vi "DATOS Y GUARDADO.vi"(6 "DATO":string, 8 "error in (no error)":errorcluster, 9 "PROVIENE DE?":enum16{"CONTADOR", "GENERADOR F"}(ring), 10 "Path":path, 11 "GUARDADOTEXTOPLANO in":refnum<class "GUARDADOTEXTOPLANO.lvclass">) -> (0 "error out":errorcluster, 3 "GUARDADOTEXTOPLANO out":refnum<class "GUARDADOTEXTOPLANO.lvclass">)   [LabVIEW 2019, in "GUARDADOTEXTOPLANO.lvlib" / "GUARDADOTEXTOPLANO.lvclass"]
uses:
  GUARDADOTEXTOPLANO.lvclass
  GUARDADOTEXTOPLANO.lvclass/GUARDADOTEXTOPLANO.ctl
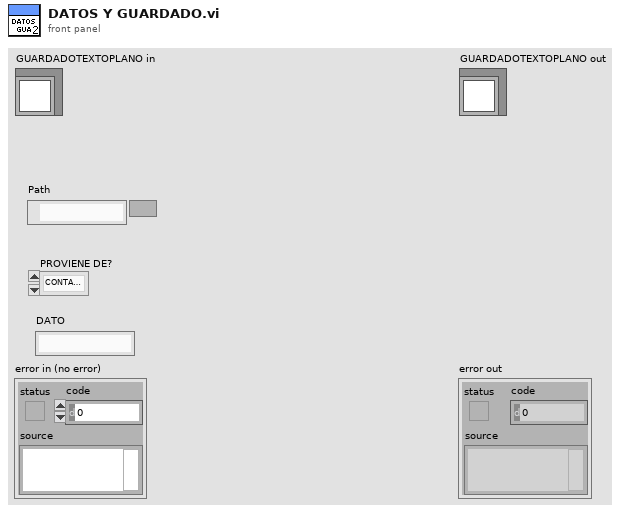
[diagram p1: front panel]
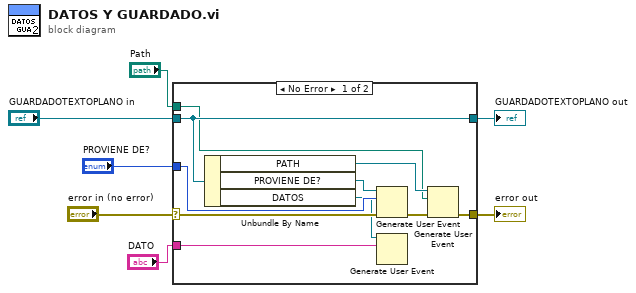
[diagram p0: block diagram]
diagram:
  n1 = case shown="No Error" "error in (no error)" {
    selector: "error in (no error)" -> [w11 w19]
    tunnel: [w10 w19] -> w6
    tunnel: [w17 w18] -> w4
    tunnel: "GUARDADOTEXTOPLANO in" -> [w17 w18]
    tunnel: "Path" -> [w14 _]
    tunnel: "PROVIENE DE?" -> [w13 _]
    tunnel: "DATO" -> [w8 _]
    frame No Error {
      n2 = Unbundle By Name(w17) -> ("PATH"=w16:refnum<user-event>, "PROVIENE DE?"=w15:refnum<user-event>, "DATOS"=w9:refnum<user-event>)
      n3 = Generate User Event(user event=w15, event data cluster=w13, error in=w11) -> (error out=w12:errorcluster)  [unwired: 1 in, 1 out]
      n4 = Generate User Event(user event=w9, event data cluster=w8) -> ()  [unwired: 2 in, 2 out]
      n5 = Generate User Event(user event=w16, event data cluster=w14, error in=w12) -> (error out=w10:errorcluster)  [unwired: 1 in, 1 out]
    }
    frame Error {
    }
  }
  "error out" <- w6
  "GUARDADOTEXTOPLANO out" <- w4
